vi "Process_Arduino_DataPacket.vi"(11 "Data Packet":string) -> (0 "error out":errorcluster, 1 "Sensor Packets Returned":i32, 2 "Sensor Readings (Signed)":i16[](array[numeric]), 3 "Time":u32)   [LabVIEW 2016]
panel:
  out "Time Packet":string
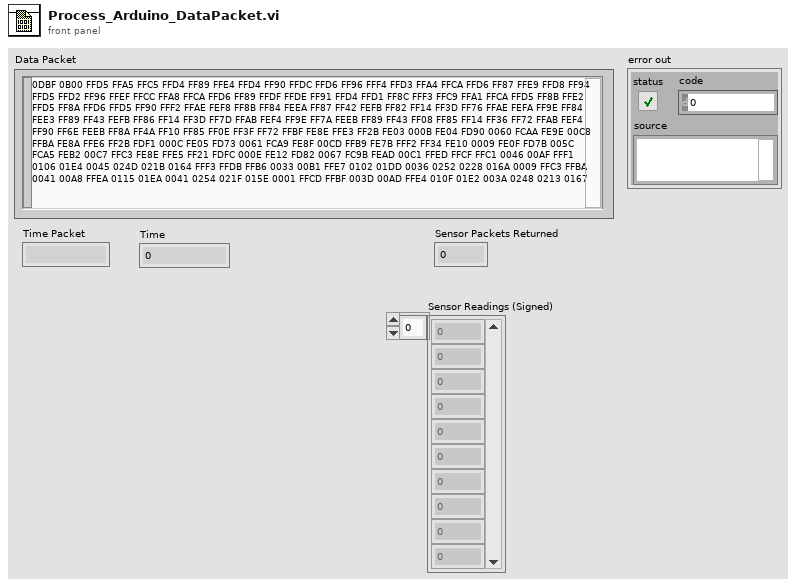
[diagram p1: front panel]
types:
  T1 = enum16{"big-endian, network order", "native, host order", "little-endian"}
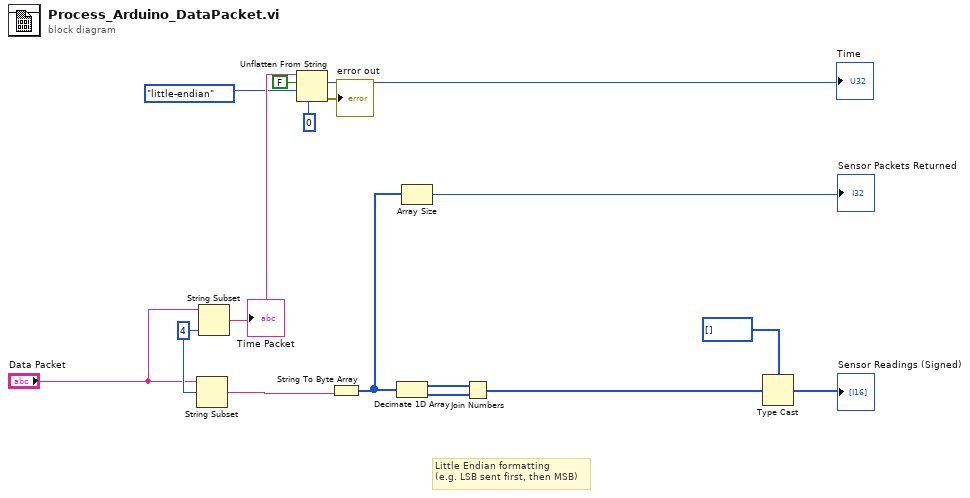
[diagram p0: block diagram]
diagram:
  w16 = 4 ("length (rest)")
  # "Little Endian formatting\n(e.g. LSB sent first, then MSB)"
  n1 = String Subset(string="Data Packet", offset (0)=w16) -> (substring=w12:string)  [unwired: 1 in]
  n2 = String Subset(string="Data Packet", length (rest)=w16) -> (substring=w15:string)  [unwired: 1 in]
  "Time Packet" <- w15
  n3 = Unflatten From String(type=u32 0 ("default (0 U32)"), binary string=w15, data includes array or string size? (T)=FALSE, byte order (0:big-endian, network order)=T1."little-endian") -> (value=→"Time":u32, error out=→"error out":errorcluster)  [unwired: 1 in, 1 out]
  n4 = String To Byte Array(string=w12) -> (unsigned byte array=w11:u8[])
  n5 = Decimate 1D Array(w11) -> (w7:u8[], w6:u8[])
  n6 = Array Size(array=w11) -> (size(s)=→"Sensor Packets Returned":i32)
  n7 = Join Numbers(hi=w7, lo=w6) -> ((hi.lo)=w4:u16[])
  n8 = Type Cast(type=i16[] [], x=w4) -> (*(type *) &x=→"Sensor Readings (Signed)":i16[])
